vi "Functional-Description.vi"() -> ()   [LabVIEW 2016, in "EV3Group10.lvrbt"]
uses:
  EV3Group10.lvrbt
  <vilib>/NXT/Block Support/NXT_InputPort.ctl
  <vilib>/NXT/Block Support/NXT_OutputPort.ctl
  <vilib>/NXT/Dual Mode Library/Display/drawText.vi
  <vilib>/NXT/Dual Mode Library/Waits/Wait_Num.vi
  <vilib>/NXT/Dual Mode Library/Sensors/EV3_Color_Reflect.vi
  <vilib>/NXT/NXTIO Xnodes/NXTIONodeSubVIs/NXTMoveMotors.vi
  <vilib>/NXT/NXTIO Xnodes/NXTIONodeSubVIs/NXTStopMotors.vi
  <vilib>/NXT/Dual Mode Library/Waits/Wait_LetGo.vi
  <vilib>/NXT/Dual Mode Library/Waits/Wait_Bump.vi
  <vilib>/NXT/Dual Mode Library/Sensors/Touch_Pressed.vi
  <vilib>/NXT/Dual Mode Library/Sensors/EV3_Ultrasonic_CM.vi
  <vilib>/NXT/NXTIO Xnodes/AddressXNode/NXTIOAddress.xnode
  <vilib>/NXT/NXTIO Xnodes/NXTIOXNode/NXTIO.xnode
  <vilib>/NXT/Subs/LVHSConnector.ctl
  <vilib>/NXT/Dual Mode Library/Waits/Wait_Touch.vi
  <vilib>/NXT/LegoClasses/BrickReference/BrickReference.lvclass
panel:
  out "Signal 2":dbl
  out "Signal 1":dbl
  out "Right Motor Speed":dbl
  out "Left Motor Speed":dbl
  out "Average Signal":dbl
  in  "Stopp":bool
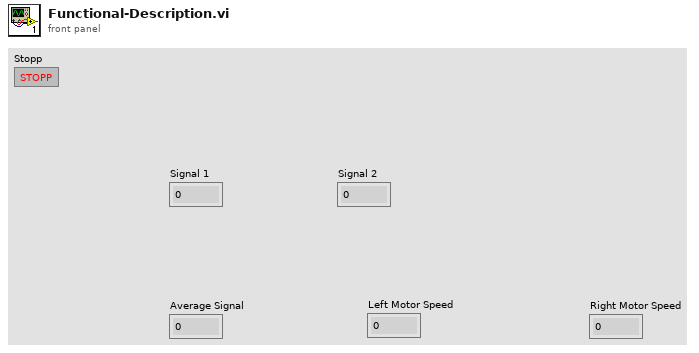
[diagram p1: front panel]
types:
  T1 = typedef "NXT_InputPort.ctl" = u32
  T2 = typedef "LVHSConnector.ctl" = refnum<class "BrickReference.lvclass">
  T3 = typedef "NXT_OutputPort.ctl" = u8
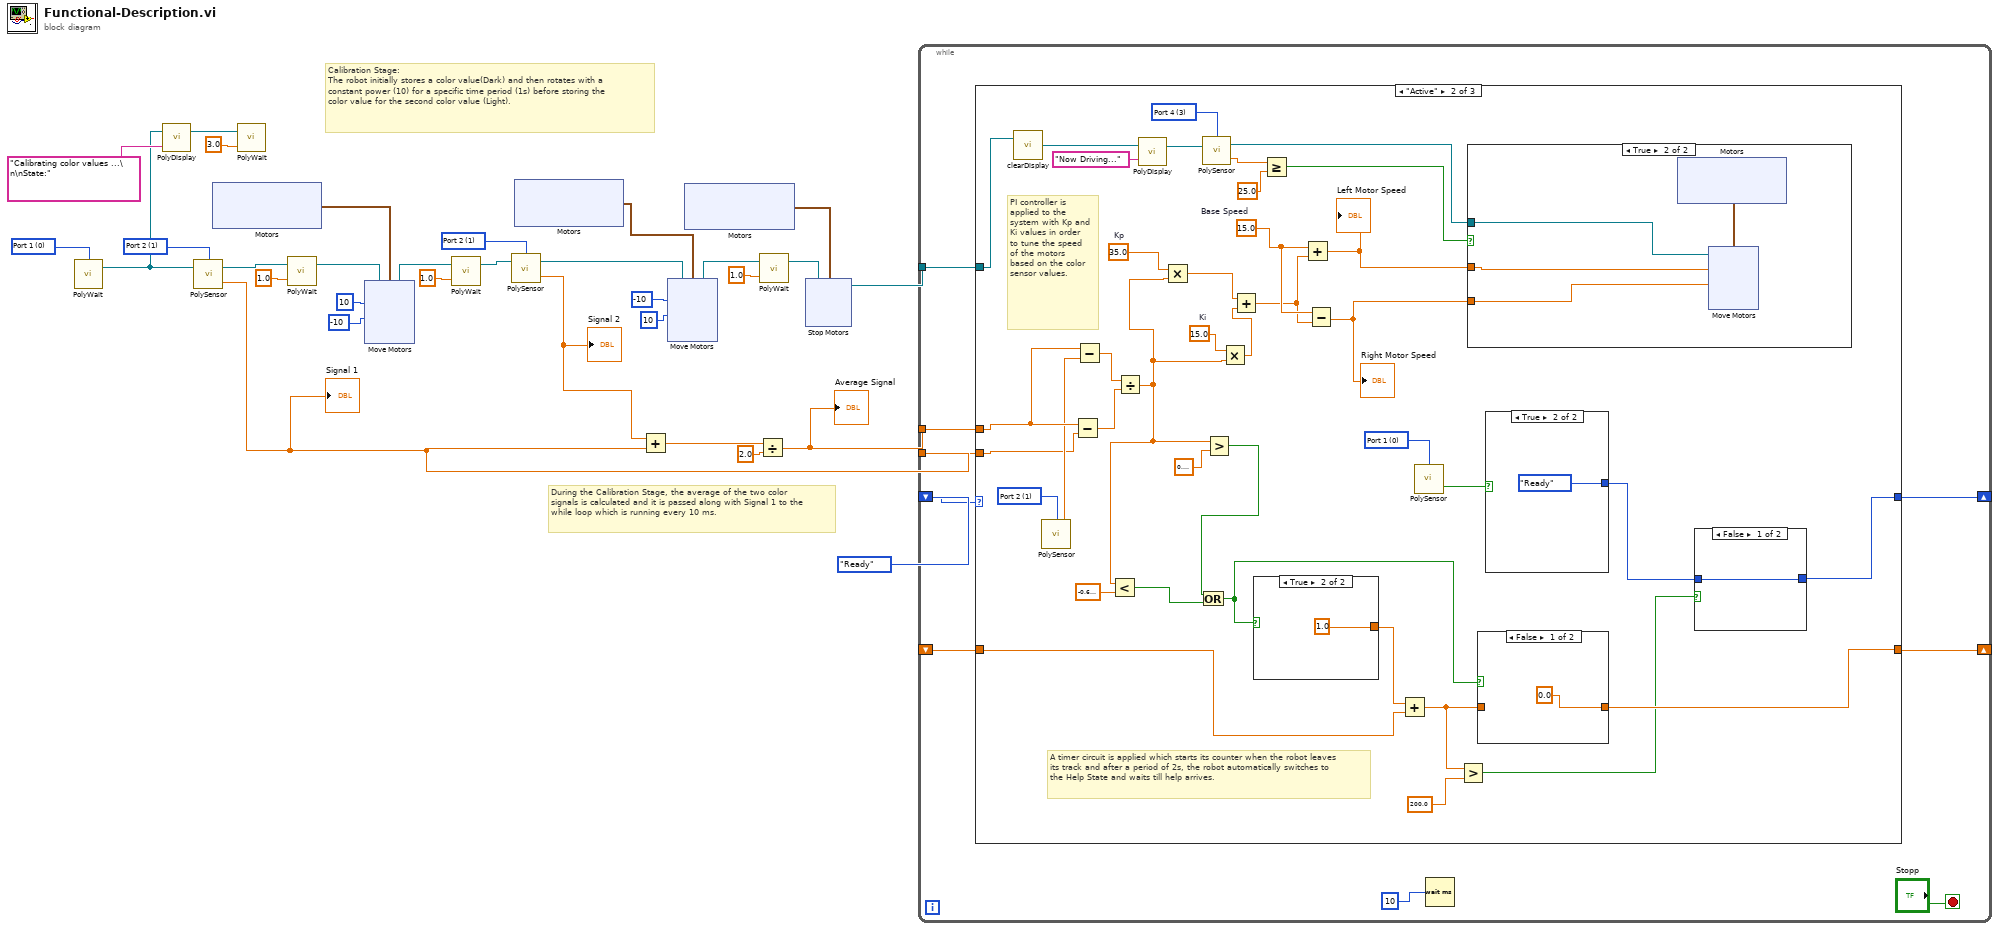
[diagram p0: block diagram]
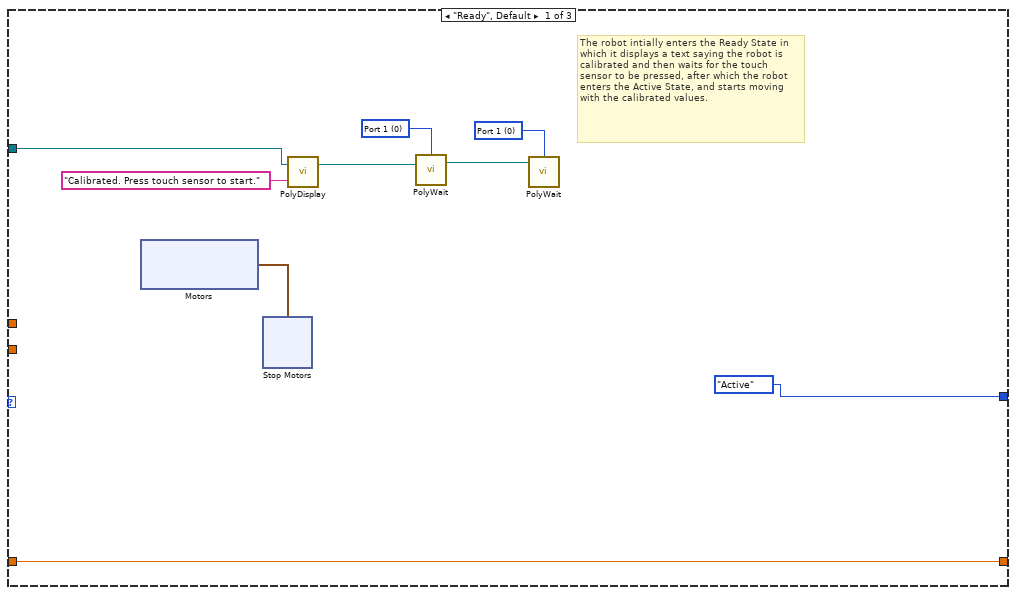
[diagram p2: hidden frame]
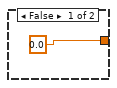
[diagram p4: hidden frame]
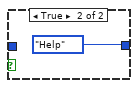
[diagram p5: hidden frame]
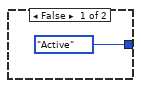
[diagram p6: hidden frame]
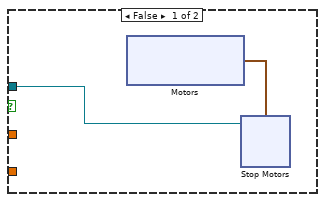
[diagram p7: hidden frame]
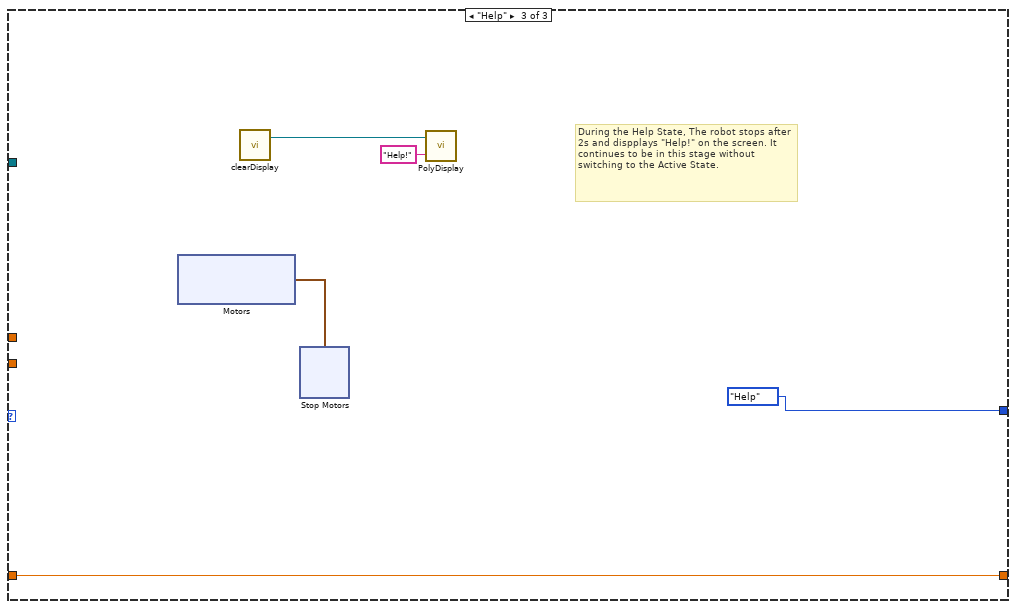
[diagram p8: hidden frame]
diagram:
  w12 = T1 1 items=["Port 1", "Port 2", "Port 3", "Port 4"] ("Port (Port 1)")
  w17 = T1 0 items=["Port 1", "Port 2", "Port 3", "Port 4"] ("Port (Port 1)")
  w31 = T1 1 items=["Port 1", "Port 2", "Port 3", "Port 4"] ("Port (Port 1)")
  # "During the Calibration Stage, the average of the two color signals is calculated and it is passed along with Signal 1 to the while loop which is running every 10 ms."
  # "Calibration Stage:\nThe robot initially stores a color value(Dark) and then rotates with a constant power (10) for a specific time period (1s) before storing the color value for the second color value (Light)."
  n1 = call-poly <vilib>:"PolyWait.vi"("Port (Port 1)"=w17) -> ("NXT/EV3"=w9:T2)  [unwired: 3 in]
  n2 = call-poly <vilib>:"PolyDisplay.vi"("Text"="Calibrating color values ...\n\nState:", "NXT/EV3"=w9) -> ("NXT/EV3"=w19:T2)  [unwired: 2 in]
  n3 = call-poly <vilib>:"PolySensor.vi"("NXT/EV3"=w9, "Port (Port 1)"=w12) -> ("Scaled Value"=w2:sgl, "NXT/EV3"=w11:T2)  [unwired: 1 in]
  "Signal 1" <- w2
  n4 = xnode "Motors"() -> ("Motor"=w30:cluster{"Port":T3, "Port":T3})
  n5 = call-poly <vilib>:"PolyWait.vi"("Time (1 sec)"=sgl 3.0, "NXT/EV3"=w19) -> ()  [unwired: 2 in, 1 out]
  n6 = call-poly <vilib>:"PolyWait.vi"("Time (1 sec)"=sgl 1.0, "NXT/EV3"=w11) -> ("NXT/EV3"=w13:T2)  [unwired: 2 in]
  n7 = xnode "Move Motors"("Power/Speed 2"=i8 -10, "Power/Speed 1"=i8 10, "Motors"=w30, "NXT/EV3"=w13) -> ("NXT/EV3"=w20:T2)
  n8 = call-poly <vilib>:"PolyWait.vi"("Time (1 sec)"=sgl 1.0, "NXT/EV3"=w20) -> ("NXT/EV3"=w16:T2)  [unwired: 2 in]
  n9 = call-poly <vilib>:"PolySensor.vi"("NXT/EV3"=w16, "Port (Port 1)"=w31) -> ("Scaled Value"=w1:sgl, "NXT/EV3"=w15:T2)  [unwired: 1 in]
  "Signal 2" <- w1
  n10 = xnode "Motors"() -> ("Motor"=w26:cluster{"Port":T3, "Port":T3})
  n11 = Add(x=w1, y=w2) -> (x+y=w8:sgl)
  n12 = xnode "Move Motors"("Power/Speed 2"=i8 10, "Power/Speed 1"=i8 -10, "Motors"=w26, "NXT/EV3"=w15) -> ("NXT/EV3"=w23:T2)
  n13 = xnode "Motors"() -> ("Motor"=w6:cluster{"Port":T3, "Port":T3})
  n14 = Divide(x=w8, y=sgl 2.0) -> (x/y=w3:sgl)
  "Average Signal" <- w3
  n15 = call-poly <vilib>:"PolyWait.vi"("Time (1 sec)"=sgl 1.0, "NXT/EV3"=w23) -> ("NXT/EV3"=w10:T2)  [unwired: 2 in]
  n16 = xnode "Stop Motors"("Motors"=w6, "NXT/EV3"=w10) -> ("NXT/EV3"=w4:T2)
  n17 = while {
    tunnel: w3 -> [w37]
    shift-right: [w34] -> _
    shift-left: _ -> [w35]
    shift-right: [w38] -> _
    shift-left: enum16{"Ready", "Active", "Help"}."Ready" -> [w33]
    tunnel: w4 -> [w39]
    tunnel: w2 -> [w32]
    stop <- "Stopp" stop-if-true
    n18 = case "Case-Struktur" shown="\"Active\"" w33 {
      tunnel: w35 -> [w49 w62 w124]
      tunnel: [w49 w59 w124] -> w34
      tunnel: w39 -> [w47 w92 _]
      tunnel: [enum16{"Ready", "Active", "Help", ""}."Active" w76 enum16{"Ready", "Active", "Help", ""}."Help"] -> w38
      tunnel: w37 -> [_ w90 _]
      tunnel: w32 -> [_ w73 _]
      frame "Ready", Default {
        w43 = T1 0 items=["Port 1", "Port 2", "Port 3", "Port 4"] ("Port (Port 1)")
        w45 = T1 0 items=["Port 1", "Port 2", "Port 3", "Port 4"] ("Port (Port 1)")
        # "The robot intially enters the Ready State in which it displays a text saying the robot is calibrated and then waits for the touch sensor to be pressed, after which the robot enters the Active State, and starts moving with the calibrated values."
        n19 = xnode "Motors"() -> ("Motor"=w42:cluster{"Port":T3, "Port":T3})
        n20 = xnode "Stop Motors"("Motors"=w42) -> ()  [unwired: 1 in, 1 out]
        n21 = call-poly <vilib>:"PolyDisplay.vi"("Text"="Calibrated. Press touch sensor to start.", "NXT/EV3"=w47) -> ("NXT/EV3"=w46:T2)  [unwired: 2 in]
        n22 = call-poly <vilib>:"PolyWait.vi"("NXT/EV3"=w46, "Port (Port 1)"=w45) -> ("NXTEV3"=w44:T2)  [unwired: 2 in]
        n23 = call-poly <vilib>:"PolyWait.vi"("NXT/EV3"=w44, "Port (Port 1)"=w43) -> ()  [unwired: 2 in, 1 out]
      }
      frame "Active" {
        w69 = sgl 15.0  # Ki
        w78 = T1 0 items=["Port 1", "Port 2", "Port 3", "Port 4"] ("Port (Port 1)")
        w87 = T1 3 items=["Port 1", "Port 2", "Port 3", "Port 4"] ("Port (Port 1)")
        w88 = sgl 15.0  # Base Speed
        w89 = sgl 35.0  # Kp
        w91 = T1 1 items=["Port 1", "Port 2", "Port 3", "Port 4"] ("Port (Port 1)")
        # "A timer circuit is applied which starts its counter when the robot leaves its track and after a period of 2s, the robot automatically switches to the Help State and waits till help arrives."
        # "PI controller is applied to the system with Kp and Ki values in order to tune the speed of the motors based on the color sensor values."
        n24 = call <vilib>:"clearDisplay.vi"("NXT/EV3"=w92) -> ("NXT/EV3"=w93:T2)  [unwired: 3 in]
        n25 = call-poly <vilib>:"PolySensor.vi"("Port (Port 1)"=w91) -> ("Scaled Value"=w74:sgl)  [unwired: 2 in, 1 out]
        n26 = Subtract(x=w90, y=w73) -> (x-y=w71:sgl)
        n27 = Subtract(x=w90, y=w74) -> (x-y=w72:sgl)
        n28 = Divide(x=w72, y=w71) -> (x/y=w65:sgl)
        n29 = Less?(x=w65, y=sgl -0.7) -> (x < y?=w64:bool)
        n30 = call-poly <vilib>:"PolyDisplay.vi"("Text"="Now Driving...", "NXT/EV3"=w93) -> ("NXT/EV3"=w86:T2)  [unwired: 2 in]
        n31 = Multiply(x=w89, y=w65) -> (x*y=w67:sgl)
        n32 = call-poly <vilib>:"PolySensor.vi"("NXT/EV3"=w86, "Port (Port 1)"=w87) -> ("Centimeters"=w85:sgl, "NXT/EV3"=w82:T2)  [unwired: 1 in]
        n33 = Greater?(x=w65, y=sgl 0.7) -> (0:w63:bool)
        n34 = Or(x=w63, y=w64) -> (x .or. y?=w60:bool)
        n35 = Multiply(x=w69, y=w65) -> (x*y=w68:sgl)
        n36 = Add(x=w67, y=w68) -> (x+y=w66:sgl)
        n37 = case shown="True" w60 {
          tunnel: [sgl 0.0 ("y") sgl 1.0 ("y")] -> w61
          frame False {
          }
          frame True {
          }
        }
        n38 = Greater Or Equal?(x=w85, y=sgl 25.0) -> (x >= y?=w83:bool)
        n39 = Add(x=w88, y=w66) -> (x+y=w80:sgl)
        "Left Motor Speed" <- w80
        n40 = Subtract(x=w88, y=w66) -> (x-y=w79:sgl)
        "Right Motor Speed" <- w79
        n41 = Add(x=w61, y=w62) -> (x+y=w58:sgl)
        n42 = call-poly <vilib>:"PolySensor.vi"("Port (Port 1)"=w78) -> ("Yes / No"=w77:bool)  [unwired: 2 in, 1 out]
        n43 = Greater?(x=w58, y=sgl 200.0) -> (0:w56:bool)
        n44 = case shown="True" w83 {
          tunnel: w80 -> [_ w113]
          tunnel: w79 -> [_ w112]
          tunnel: w82 -> [w103 w111]
          frame False {
            n45 = xnode "Motors"() -> ("Motor"=w104:cluster{"Port":T3, "Port":T3})
            n46 = xnode "Stop Motors"("Motors"=w104, "NXT/EV3"=w103) -> ()  [unwired: 1 out]
          }
          frame True {
            n47 = xnode "Motors"() -> ("Motor"=w114:cluster{"Port":T3, "Port":T3})
            n48 = xnode "Move Motors"("Power/Speed 2"=w112, "Power/Speed 1"=w113, "Motors"=w114, "NXT/EV3"=w111) -> ()  [unwired: 1 out]
          }
        }
        n49 = case shown="False" w60 {
          tunnel: w58 -> [_ w96]
          tunnel: [sgl 0.0 ("y") w96] -> w59
          frame False {
          }
          frame True {
          }
        }
        n50 = case shown="True" w77 {
          tunnel: [enum16{"Ready", "Active", "Help", ""}."Active" enum16{"Ready", "Active", "Help", ""}."Ready"] -> w70
          frame False {
          }
          frame True {
          }
        }
        n51 = case shown="False" w56 {
          tunnel: [w99 enum16{"Ready", "Active", "Help", ""}."Help"] -> w76
          tunnel: w70 -> [w99 _]
          frame False {
          }
          frame True {
          }
        }
      }
      frame "Help" {
        # "During the Help State, The robot stops after 2s and dispplays \"Help!\" on the screen. It continues to be in this stage without switching to the Active State."
        n52 = xnode "Motors"() -> ("Motor"=w128:cluster{"Port":T3, "Port":T3})
        n53 = call <vilib>:"clearDisplay.vi"() -> ("NXT/EV3"=w127:T2)  [unwired: 4 in]
        n54 = xnode "Stop Motors"("Motors"=w128) -> ()  [unwired: 1 in, 1 out]
        n55 = call-poly <vilib>:"PolyDisplay.vi"("Text"="Help!", "NXT/EV3"=w127) -> ()  [unwired: 2 in, 1 out]
      }
    }
    n56 = Wait (ms)(milliseconds to wait=u32 10 ("Zu wartende ms")) -> ()  [unwired: 1 out]
  }
